vi "Register Configuration and Results.vi"(8 "error in (no error)":errorcluster, 10 "Measurement":refnum<class "MeasurementPluginService.lvclass">, 11 "gRPC ID":T1) -> (0 "error out":errorcluster, 3 "gRPC ID Out":T1)   [LabVIEW 2020, in "MeasurementLink Measurement Server.lvlib"]
uses:
  MeasurementLink Measurement Server.lvlib
  <vilib>/gRPC/LabVIEW gRPC Library/Shared/grpcId.ctl
  Classes/MeasurementPluginService/MeasurementPluginService.lvclass
  <vilib>/gRPC/LabVIEW gRPC Library/grpc-lvsupport-release.lvlib
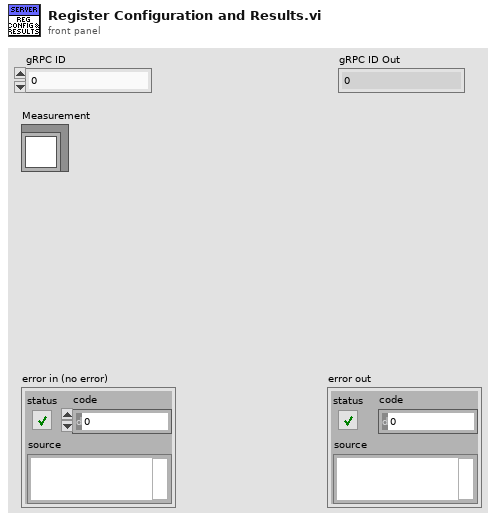
[diagram p1: front panel]
types:
  T1 = typedef "grpc-lvsupport-release.lvlib/grpcId.ctl" = u64
  T2 = typedef "grpc-lvsupport-release.lvlib/Message Metadata.ctl" = cluster{"Version":i32, "Name":string, "Type Url":string, "Elements":T3[]}
  T3 = typedef "grpc-lvsupport-release.lvlib/Message Element Metadata.ctl" = cluster{"Embedded Message Name":string, "Protobuf Index":i32, "MessageElementType":T4, "Repeated":bool}
  T4 = typedef "grpc-lvsupport-release.lvlib/Message Element Type.ctl" = enum32{"Int32Value", "FloatValue", "DoubleValue", "BoolValue", "StringValue", "MessageValue", "Int64Value", "UInt32Value", "UInt64Value", "EnumValue", "Bytes", "Fixed64", "Fixed32", "SFixed64", "SFixed32", "SInt64", "SInt32"}
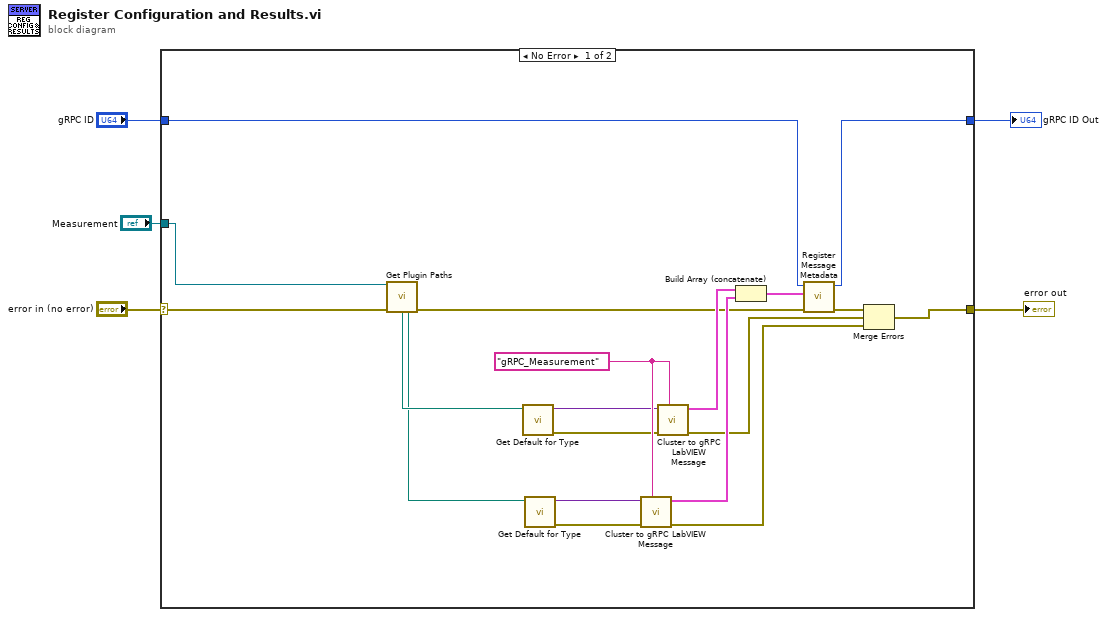
[diagram p0: block diagram]
diagram:
  n1 = case shown="No Error" "error in (no error)" {
    selector: "error in (no error)" -> [w9 w26]
    tunnel: [w17 w25] -> w2
    tunnel: [w20 w26] -> w5
    tunnel: "gRPC ID" -> [w16 w25]
    tunnel: "Measurement" -> [w10 _]
    frame No Error {
      w15 = "gRPC_Measurement" ("Package Name")
      n2 = call-dynamic "Get Plugin Paths.vi"("MeasurementService in"=w10, "error in (no error)"=w9) -> ("Measurement Configuration CTL Path"=w7:path, "Measurement Results CTL Path"=w6:path, "error out"=w8:errorcluster)  [unwired: 7 in, 4 out]
      n3 = call "Get Default for Type.vi"("Path of Type"=w7) -> ("error out"=w13:errorcluster, "Default for Type"=w14:variant)  [unwired: 9 in]
      n4 = call "Get Default for Type.vi"("Path of Type"=w6) -> ("error out"=w11:errorcluster, "Default for Type"=w12:variant)  [unwired: 9 in]
      n5 = call <vilib>:"Cluster to gRPC LabVIEW Message.vi"("Package Name"=w15, "error in"=w11, "Cluster"=w12) -> ("error out"=w19:errorcluster, "gRPC Message Metadata []"=w22:T2[])  [unwired: 7 in]
      n6 = call <vilib>:"Cluster to gRPC LabVIEW Message.vi"("Package Name"=w15, "error in"=w13, "Cluster"=w14) -> ("error out"=w18:errorcluster, "gRPC Message Metadata []"=w23:T2[])  [unwired: 7 in]
      n7 = Build Array (concatenate)(w23, w22) -> (w21:T2[])
      n8 = call <vilib>:"Register Message Metadata.vi"("error in"=w8, "Messages"=w21, "gRPCid in"=w16) -> ("error out"=w24:errorcluster, "gRPCid out"=w17:T1)  [unwired: 7 in]
      n9 = Merge Errors(w24, w18, w19) -> (w20:errorcluster)
    }
    frame Error {
    }
  }
  "error out" <- w5
  "gRPC ID Out" <- w2
